vi "MUX Selection Dialog.vi"(8 "error in (no error)":errorcluster, 10 "Current selection":string, 11 "NIVS.System Definition Root":refnum<k24>) -> (0 "error out":errorcluster, 1 "Cancelled":bool, 2 "New selection":string)   [LabVIEW 2013]
doc: "Use this template to create a dialog box with event handling."
uses:
  NationalInstruments.VeriStand.SystemStorageUI
  NationalInstruments.VeriStand.SystemStorage
  NationalInstruments.VeriStand
  <vilib>/NI Veristand/UI Controls/Single Node Browser/NI_VS UI Single Node Browser.lvlib
panel:
  in  "Cancel":bool
  in  "Ok":bool
  in  "Selected MUX":refnum<k24>(container)
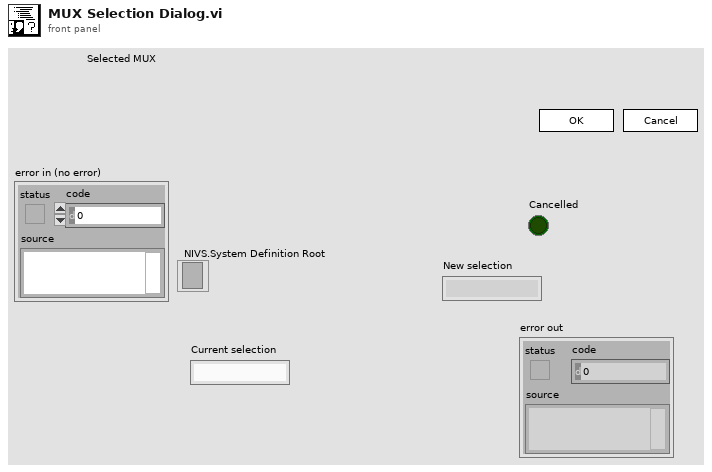
[diagram p1: front panel]
types:
  T1 = typedef "NI_VS UI Single Node Browser.lvlib/Callback Type.ctl" = cluster{"Net Callbacks":refnum<k27>[], "Event":refnum<user-event>}
  T2 = typedef "NI_VS UI Single Node Browser.lvlib/Node Ref.ctl" = refnum<k24>
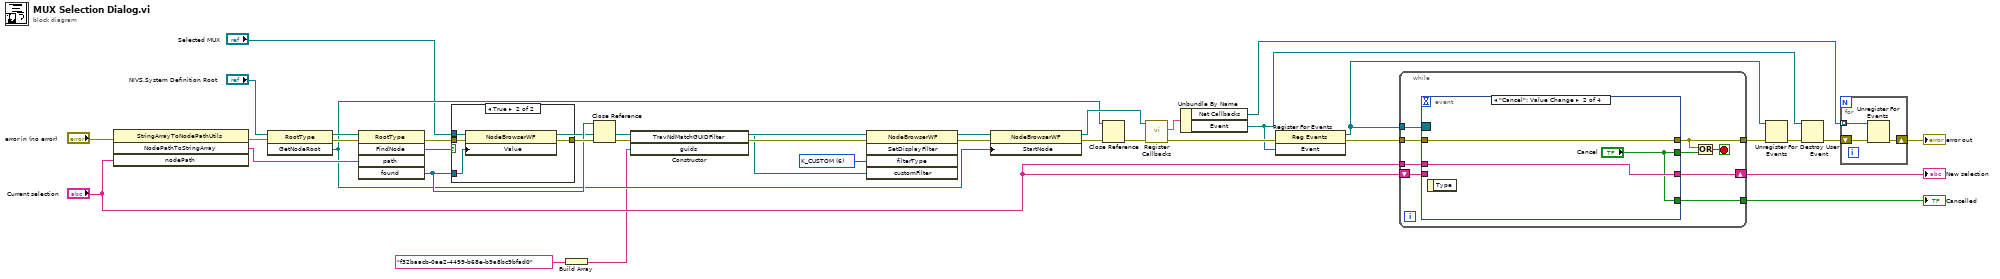
[diagram p0: block diagram]
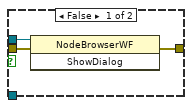
[diagram p2: hidden frame]
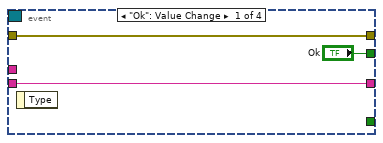
[diagram p3: hidden frame]
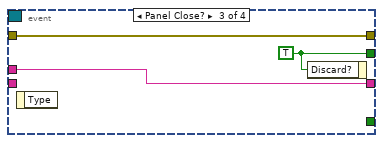
[diagram p4: hidden frame]
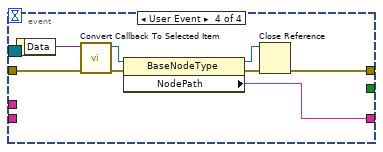
[diagram p5: hidden frame]
diagram:
  w5 = u8 6 items=["K_CHAN_R", "K_CHAN_W", "K_CHAN_RW", "K_CHAN_VOLT", "K_CHAN_FAULT", "K_ALL", "K_CUSTOM", "K_CHAN_R_VIS", "K_CHAN_W_VIS", "K_CHAN_RW_VIS", "K_CHAN_VOLT_VIS", "K_CHAN_FAULT_VIS", "K_WAVE", "K_WAVE_VIS", "K_WAVE_DBL", "K_WAVE_CDB", "K_WAVE_DBL_VIS", "K_WAVE_CDB_VIS"] ("filterType")
  n1 = invoke class="StringArrayToNodePathUtils" method="NodePathToStringArray"(error in="error in (no error)", "nodePath"="Current selection") -> (error out=w16:errorcluster, "NodePathToStringArray"=w15:string[])  [unwired: 2 in, 2 out]
  n2 = invoke class="RootType" method="GetNodeRoot"(reference="NIVS.System Definition Root", error in=w16) -> (reference out=w34:refnum<k24>, error out=w35:errorcluster, "GetNodeRoot"=w11:refnum<k24>)  [unwired: 1 in]
  n3 = invoke class="RootType" method="FindNode"(reference=w34, error in=w35, "path"=w15) -> (error out=w30:errorcluster, "FindNode"=w29:bool, "found"=w13:refnum<k24>)  [unwired: 2 in, 2 out]
  n4 = case shown="True" w29 {
    tunnel: w13 -> [_ w41]
    tunnel: w30 -> [w39 w42]
    tunnel: [w37 w40] -> w26
    tunnel: "Selected MUX" -> [w38 w43]
    frame False {
      n5 = invoke class="NodeBrowserWF" method="ShowDialog"(reference=w38, error in=w39) -> (error out=w37:errorcluster)  [unwired: 1 in, 2 out]
    }
    frame True {
      n6 = property class="NodeBrowserWF"(reference=w43, error in=w42, "Value"=w41) -> (error out=w40:errorcluster)  [unwired: 1 out]
    }
  }
  n7 = Build Array("f32baacb-0ae2-4499-b68e-b9a8bc9bfad0") -> (w6:string[])
  n8 = Close Reference(reference=w13, error in (no error)=w26) -> (error out=w4:errorcluster)
  n9 = constructor class="TravNdMatchGUIDFilter"(error in=w4, "guids"=w6) -> (reference out=w2:refnum<k24>, error out=w3:errorcluster)  [unwired: 2 in, 2 out]
  n10 = invoke class="NodeBrowserWF" method="SetDisplayFilter"(reference="Selected MUX", error in=w3, "filterType"=w5, "customFilter"=w2) -> (reference out=w8:refnum<k24>, error out=w1:errorcluster)  [unwired: 1 in, 3 out]
  n11 = property class="NodeBrowserWF"(reference=w8, error in=w1, "StartNode"=w11) -> (reference out=w31:refnum<k24>, error out=w32:errorcluster)
  n12 = Close Reference(reference=w11, error in (no error)=w32) -> (error out=w12:errorcluster)
  n13 = call <vilib>:"Register Callbacks.vi"("error in (no error)"=w12, "Single Node Browser"=w31) -> ("error out"=w36:errorcluster, "Callbacks"=w33:T1)  [unwired: 7 in, 1 out]
  n14 = Unbundle By Name(w33) -> ("Net Callbacks"=w21:refnum<k27>[], "Event"=w20:refnum<user-event>)
  n15 = register-events(error in=w36, w20) -> (reference out=w23:refnum<event-registration>, error out=w27:errorcluster)  [unwired: 1 in]
  n16 = while {
    tunnel: [w45] -> w25
    tunnel: w27 -> [w51]
    tunnel: w23 -> [w49]
    shift-right: [w48] -> w28
    shift-left: "Current selection" -> [w47]
    tunnel: "Current selection" -> [w46]
    tunnel: [w44] -> w10
    stop <- w50 stop-if-true
    n17 = event shown="[1] \"Cancel\": Value Change" {
      selector: w49 -> [_ _ _ _]
      dyn-events: _ -> [_ _ _ _]
      timeout: _ -> [_ _ _ _]
      tunnel: ["Ok" "Cancel" w61 _] -> w52
      tunnel: [w55 w58 w60 w67] -> w45
      tunnel: w51 -> [w55 w58 w60 w68]
      tunnel: [w53 w57 w59 w62] -> w48
      tunnel: w47 -> [w53 _ _ _]
      tunnel: w46 -> [_ w57 w59 _]
      tunnel: [_ "Cancel" _ _] -> w44
      event "Ok": Value Change {
        n18 = event-data() -> ()  [unwired: 1 in, 1 out]
      }
      event "Cancel": Value Change {
        n19 = event-data() -> ()  [unwired: 1 in, 1 out]
      }
      event Panel Close? {
        w61 = TRUE ("Cancel")
        n20 = event-data() -> ()  [unwired: 1 in, 1 out]
        n21 = event-data("Discard?"=w61) -> ()  [unwired: 1 in, 1 out]
      }
      event User Event {
        n22 = event-data() -> ("Data"=w69:variant)  [unwired: 1 in]
        n23 = call <vilib>:"Convert Callback To Selected Item.vi"("error in"=w68, "Data"=w69) -> ("error out"=w63:errorcluster, "Selected Item"=w66:T2)  [unwired: 8 in]
        n24 = property class="BaseNodeType"(reference=w66, error in=w63) -> (reference out=w65:T2, error out=w64:errorcluster, "NodePath"=w62:string)
        n25 = Close Reference(reference=w65, error in (no error)=w64) -> (error out=w67:errorcluster)
      }
    }
    n26 = Or(x=w45, y=w52) -> (x .or. y?=w50:bool)
  }
  "New selection" <- w28
  "Cancelled" <- w10
  n27 = Unregister For Events(event registration refnum=w23, error in=w25) -> (error out=w24:errorcluster)
  n28 = Destroy User Event(user event=w20, error in=w24) -> (error out=w22:errorcluster)
  n29 = for {
    tunnel: w21 -> [w71] mode=indexing
    shift-right: [w70] -> w14
    shift-left: w22 -> [w72]
    n30 = Unregister For Events(event registration refnum=w71, error in=w72) -> (error out=w70:errorcluster)
  }
  "error out" <- w14
